vi "ROI entry-Get experiment folder path.vi"(8 "error in (no error)":errorcluster) -> (0 "error out":errorcluster, 3 "Experiment folder path":path)   [LabVIEW 2017]
uses:
  ROI Entry screen/Globals/gl_ROI Entry UI globals.vi
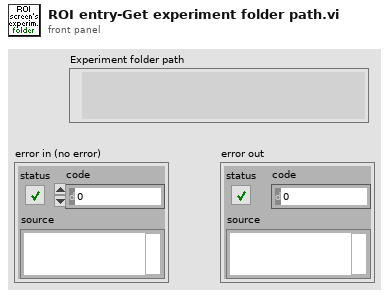
[diagram p1: front panel]
types:
  T1 = typedef "ROI entry screen ctrl refs cluster.ctl" = cluster{"Done button":refnum<vi>, "Imaging button":refnum<vi>, "Acquisition button":refnum<vi>, "POI dwell time (us)":refnum<vi>, "Scan dwell time per pixel (us)":refnum<vi>, "# of planes":refnum<vi>, "Zoom Ctrl":refnum<vi>, "Equal size":refnum<vi>, "Channel":refnum<vi>, "Image Display":refnum<vi>, "Z-Plane Selector":refnum<vi>, "Number of lines left":refnum<vi>, "Z-stack folder path":refnum<vi>, "POI Density":refnum<vi>, "Arb Plane Entry":refnum<vi>, "Whole plane":refnum<vi>, "Clear Last":refnum<vi>, "Clear All":refnum<vi>, "Trial Length (sec)":refnum<vi>, "Palette Type":refnum<vi>, "Intensity slider":refnum<vi>, "# POI":refnum<vi>, "Max Z Proj":refnum<vi>, "Zplane ind":refnum<vi>, "Wavelength (nm)":refnum<vi>, "Number of Trials":refnum<vi>, "Funct stim.trig.enable":refnum<vi>, "Funct stim.trig.delay (s)":refnum<vi>, "Line Mode":refnum<vi>, "Step size (µm)":refnum<vi>, "ROI move mode":refnum<vi>, "Cool-down time (s)":refnum<vi>, "Enable cool-down time":refnum<vi>, "Motor Z ind. (um)":refnum<vi>, "AOL Z ind. (um)":refnum<vi>, "Load Reference Image":refnum<vi>}
  T2 = typedef "Fixed strings.ctl" = cluster{"ROI file name":string, "Normalised ROI file name":string, "Zplane Pockels values file name":string, "Functional data folder name":string, "Experiment Header file name":string, "Z-stack images folder name":string, "Groups setup rel. path":string, "Groups text file rel. path":string, "TDMS files folder name (F.img)":string, "TDMS files folder name (V.acq)":string, "TDMS files folder name (Pl.acq)":string, "Cycle rel times sequence file":string, "Dynamically called VIs folder name":string, "Time Series folder base name":string}
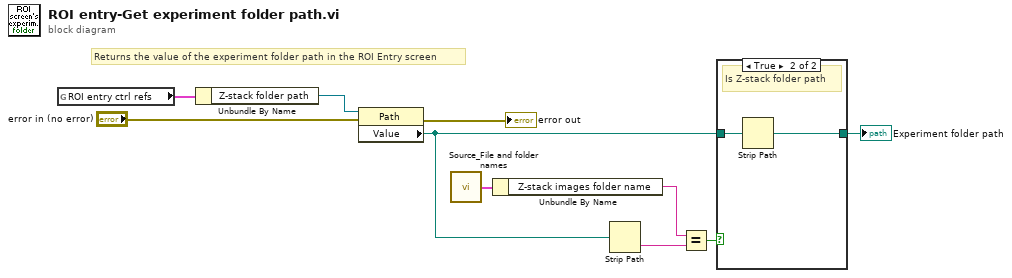
[diagram p0: block diagram]
diagram:
  # "Returns the value of the experiment folder path in the ROI Entry screen"
  n1 = global read "gl_ROI Entry UI globals.vi" "ROI entry ctrl refs"() -> (w10:T1)
  n2 = Unbundle By Name(w10) -> ("Z-stack folder path"=w9:refnum<vi>)
  n3 = property on="Property Node" class="Path"(reference=w9, error in="error in (no error)") -> (error out=→"error out":errorcluster, "Value"=w2:path)  [unwired: 1 out]
  n4 = call "Source_File and folder names.vi"() -> ("Fixed strings"=w5:T2)  [unwired: 1 in]
  n5 = Unbundle By Name(w5) -> ("Z-stack images folder name"=w4:string)
  n6 = Strip Path(path=w2) -> (name=w6:string)  [unwired: 1 out]
  n7 = Equal?(x=w4, y=w6) -> (x = y?=w3:bool)
  n8 = case shown="True" w3 {
    tunnel: w2 -> [w11 w13]
    tunnel: [w11 w12] -> w1
    frame False {
      # "Is not Z-stack folder path"
    }
    frame True {
      # "Is Z-stack folder path"
      n9 = Strip Path(path=w13) -> (stripped path=w12:path)  [unwired: 1 out]
    }
  }
  "Experiment folder path" <- w1
